vi "Calculate Chunk string size.vi"(0 "String":string, 5 "Font":T2={"Name"="", "Size"=12.0, "Color"=0, "Style"={"Bold"=FALSE, "Italic"=FALSE, "Underline"=FALSE, "Strikeout"=FALSE}}, 7 "Font refnum":refnum<k24>, 9 "System Fonts":T1, 11 "error in (no error)":errorcluster) -> (4 "DescentPoint":sgl, 6 "Width":sgl, 10 "Height":sgl, 15 "error out":errorcluster)   [LabVIEW 2013]
doc: "Version 1.0\nDeveloped by Jean-Marc Simard\nCopyright © 2010, Exaprom Inc.\nAll rights reserved.\nLicense: BSD\n\nWith iTextSharp 4.1.6 (http://itextsharp.sourceforge.net)\nunder Mozilla Public License Version 1.1\n(http://www.mozilla.org/MPL/MPL-1.1.html)"
uses:
  Controls/Font cluster.ctl
  Controls/Font size.ctl
  Controls/Font color.ctl
  Controls/System Fonts.ctl
  C:/Users/MaxCorp/Documents/GitHub/TopView/DLL/itextsharp.dll
  DLL/itextsharp.dll
panel:
  out "x-y":u32
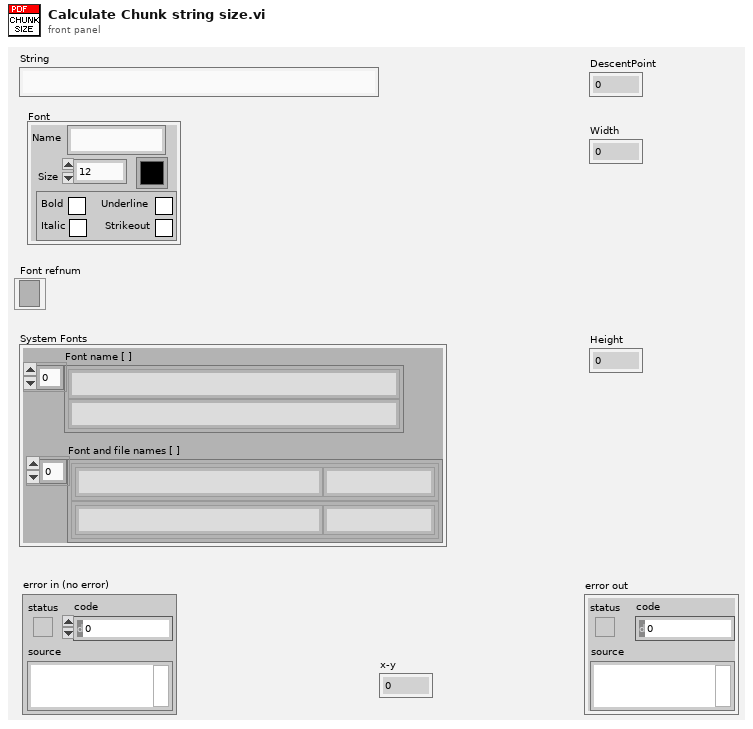
[diagram p1: front panel]
types:
  T1 = typedef "System Fonts.ctl" = cluster{"Font name [ ]":string[], "Font and file names [ ]":cluster{"Font name":string, "File name":string}[]}
  T2 = typedef "Font cluster.ctl" = cluster{"Name":string, "Size":T3, "Color":T4, "Style":cluster{"Bold":bool, "Italic":bool, "Underline":bool, "Strikeout":bool}}
  T3 = typedef "Font size.ctl" = sgl
  T4 = typedef "Font color.ctl" = u32
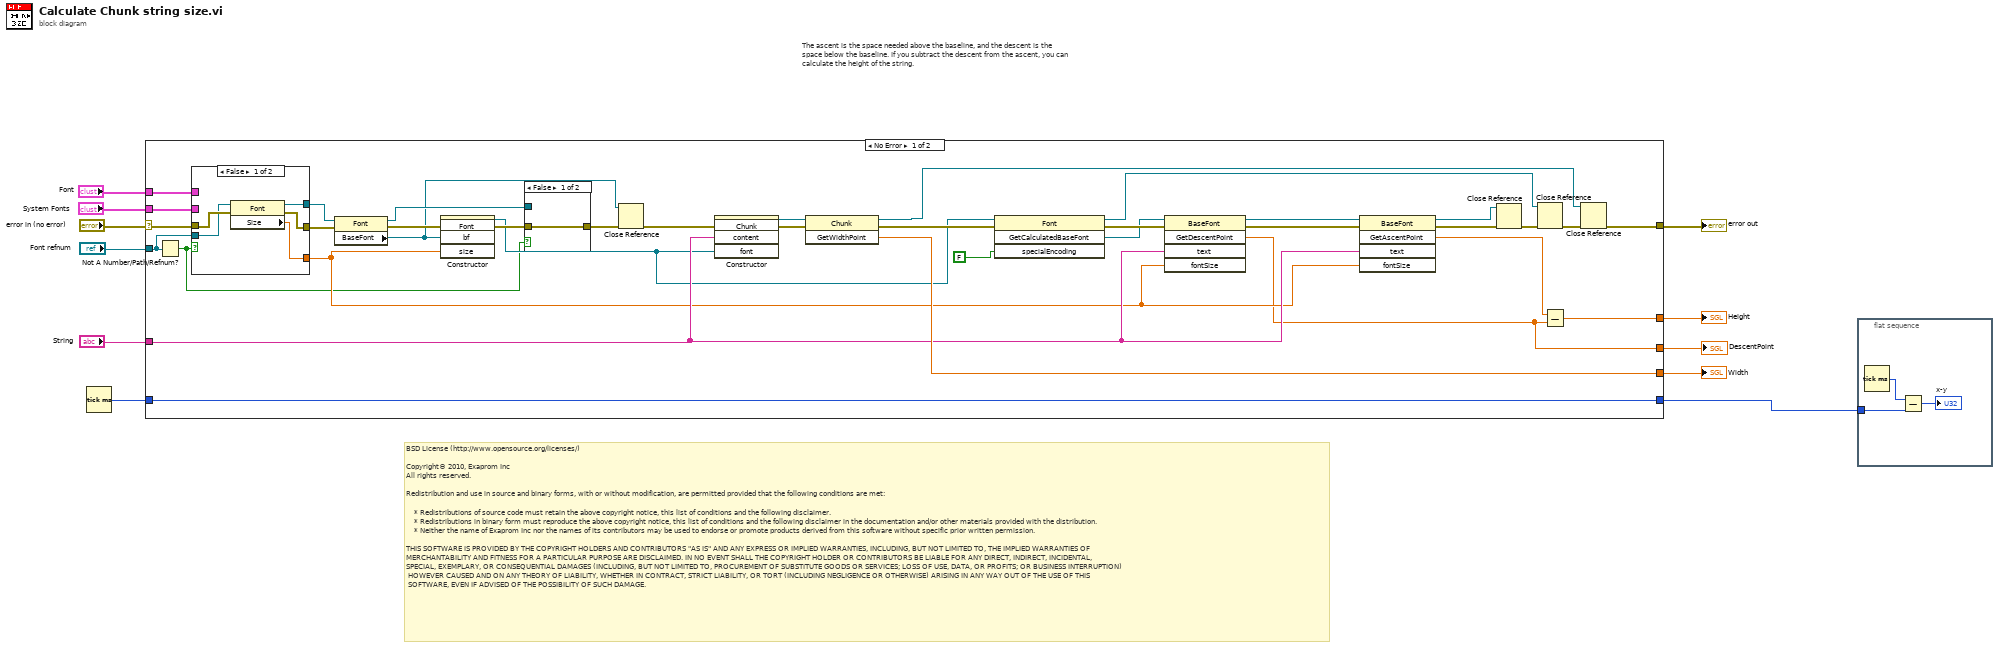
[diagram p0: block diagram]
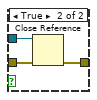
[diagram p2: hidden frame]
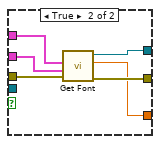
[diagram p3: hidden frame]
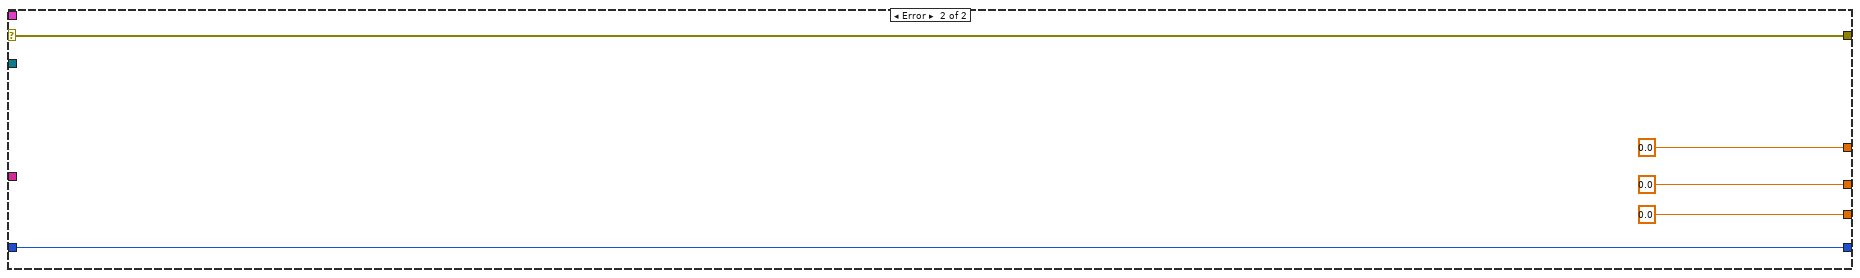
[diagram p4: hidden frame]
diagram:
  # "The ascent is the space needed above the baseline, and the descent is the\nspace below the baseline. If you subtract the descent from the ascent, you can\ncalculate the height of the string."
  # "BSD License (http://www.opensource.org/licenses/)\n\nCopyright© 2010, Exaprom Inc\nAll rights reserved.\n\nRedistribution and use in source and binary forms, with or without modification, are permitted provided that the following conditions are met:\n\n    * Redistributions of source code must retain the above copyright notice, this list of conditions and the following disclaimer.\n    * Redistributions in binary form must reproduce the above copyright notice, this list of conditions and the following disclaimer in the documentation and/or other materials provided with the distribution.\n    * Neither the name of Exaprom Inc nor the names of its contributors may be used to endorse or promote products derived from this software without specific prior written permission.\n\nTHIS SOFTWARE IS PROVIDED BY THE COPYRIGHT HOLDERS AND CONTRIBUTORS \"AS IS\" AND ANY EXPRESS OR IMPLIED WARRANTIES, INCLUDING, BUT NOT LIMITED TO, THE IMPLIED WARRANTIES OF \nMERCHANTABILITY AND FITNESS FOR A PARTICULAR PURPOSE ARE DISCLAIMED. IN NO EVENT SHALL THE COPYRIGHT HOLDER OR CONTRIBUTORS BE LIABLE FOR ANY DIRECT, INDIRECT, INCIDENTAL,\nSPECIAL, EXEMPLARY, OR CONSEQUENTIAL DAMAGES (INCLUDING, BUT NOT LIMITED TO, PROCUREMENT OF SUBSTITUTE GOODS OR SERVICES; LOSS OF USE, DATA, OR PROFITS; OR BUSINESS INTERRUPTION)\n HOWEVER CAUSED AND ON ANY THEORY OF LIABILITY, WHETHER IN CONTRACT, STRICT LIABILITY, OR TORT (INCLUDING NEGLIGENCE OR OTHERWISE) ARISING IN ANY WAY OUT OF THE USE OF THIS\n SOFTWARE, EVEN IF ADVISED OF THE POSSIBILITY OF SUCH DAMAGE."
  n1 = Tick Count (ms)() -> (millisecond timer value=w3:u32)
  n2 = case shown="No Error" "error in (no error)" {
    selector: "error in (no error)" -> [w27 w67]
    tunnel: [w44 sgl 0.0 ("GetWidthPoint")] -> w11
    tunnel: [w43 sgl 0.0] -> w10
    tunnel: "String" -> [w34 _]
    tunnel: [w33 w67] -> w8
    tunnel: "Font" -> [w29 _]
    tunnel: [w24 sgl 0.0 ("GetDescentPoint")] -> w5
    tunnel: "System Fonts" -> [w26 _]
    tunnel: [w25 w63] -> w2
    tunnel: w3 -> [w25 w63]
    tunnel: "Font refnum" -> [w13 _]
    frame No Error {
      n3 = Not A Number/Path/Refnum?(number/path/refnum=w13) -> (NaN/Path/Refnum?=w12:bool)
      n4 = case shown="False" w12 {
        tunnel: [w52 w62] -> w32
        tunnel: [w54 w61] -> w31
        tunnel: [w53 w60] -> w30
        tunnel: w29 -> [_ w59]
        tunnel: w27 -> [w56 w58]
        tunnel: w26 -> [_ w57]
        tunnel: w13 -> [w55 _]
        frame False {
          n5 = property class="Font"(reference=w55, error in=w56) -> (reference out=w52:refnum<k24>, error out=w54:errorcluster, "Size"=w53:sgl)
        }
        frame True {
          n6 = call "Get Font.vi"("error in (no error)"=w58, "System Fonts"=w57, "Font IN"=w59) -> ("error out"=w61:errorcluster, "Font Size"=w60:T3, "Font"=w62:refnum<k24>)  [unwired: 6 out]
        }
      }
      n7 = property class="Font"(reference=w32, error in=w31) -> (reference out=w23:refnum<k24>, error out=w22:errorcluster, "BaseFont"=w16:refnum<k24>)
      n8 = constructor class="Font"(error in=w22, "bf"=w16, "size"=w30) -> (reference out=w15:refnum<k24>, error out=w21:errorcluster)  [unwired: 2 in, 3 out]
      n9 = case shown="False" w12 {
        tunnel: w23 -> [_ w51]
        tunnel: w21 -> [w48 w50]
        tunnel: [w48 w49] -> w18
        frame False {
        }
        frame True {
          n10 = Close Reference(reference=w51, error in (no error)=w50) -> (error out=w49:errorcluster)
        }
      }
      n11 = Close Reference(reference=w16, error in (no error)=w18) -> (error out=w17:errorcluster)
      n12 = constructor class="Chunk"(error in=w17, "content"=w34, "font"=w15) -> (reference out=w19:refnum<k24>, error out=w20:errorcluster)  [unwired: 2 in, 3 out]
      n13 = invoke class="Chunk" method="GetWidthPoint"(reference=w19, error in=w20) -> (reference out=w35:refnum<k24>, error out=w40:errorcluster, "GetWidthPoint"=w44:sgl)  [unwired: 1 in]
      n14 = invoke class="Font" method="GetCalculatedBaseFont"(reference=w15, error in=w40, "specialEncoding"=FALSE) -> (reference out=w37:refnum<k24>, error out=w42:errorcluster, "GetCalculatedBaseFont"=w28:refnum<k24>)  [unwired: 1 in, 1 out]
      n15 = invoke class="BaseFont" method="GetDescentPoint"(reference=w28, error in=w42, "text"=w34, "fontSize"=w30) -> (reference out=w46:refnum<k24>, error out=w45:errorcluster, "GetDescentPoint"=w24:sgl)  [unwired: 1 in, 2 out]
      n16 = invoke class="BaseFont" method="GetAscentPoint"(reference=w46, error in=w45, "text"=w34, "fontSize"=w30) -> (reference out=w14:refnum<k24>, error out=w39:errorcluster, "GetAscentPoint"=w41:sgl)  [unwired: 1 in, 2 out]
      n17 = Close Reference(reference=w14, error in (no error)=w39) -> (error out=w38:errorcluster)
      n18 = Close Reference(reference=w37, error in (no error)=w38) -> (error out=w36:errorcluster)
      n19 = Subtract(x=w41, y=w24) -> (x-y=w43:sgl)
      n20 = Close Reference(reference=w35, error in (no error)=w36) -> (error out=w33:errorcluster)
    }
    frame Error {
    }
  }
  "Width" <- w11
  "Height" <- w10
  "error out" <- w8
  "DescentPoint" <- w5
  n21 = flat-sequence {
    tunnel: w2 -> [w69]
    frame #0 {
      n22 = Tick Count (ms)() -> (millisecond timer value=w70:u32)
      n23 = Subtract(x=w70, y=w69) -> (x-y=→"x-y":u32)
    }
  }
